vi "Prompt for Step--Update State Data.vi"(8 "error in (no error)":errorcluster, 9 "Data":variant, 10 "Argument":string, 11 "Keyboard Action in":refnum<class "Keyboard Action.lvclass">) -> (0 "error out":errorcluster, 3 "Keyboard Action out":refnum<class "Keyboard Action.lvclass">)   [LabVIEW 2020, in "MacroAssert.lvlib" / "Keyboard Action.lvclass"]
uses:
  Keyboard Action.lvclass
  Keyboard Action.lvclass/Keyboard Action.ctl
  Keyboard Action Type.ctl
  Action Step/Action Step.lvclass
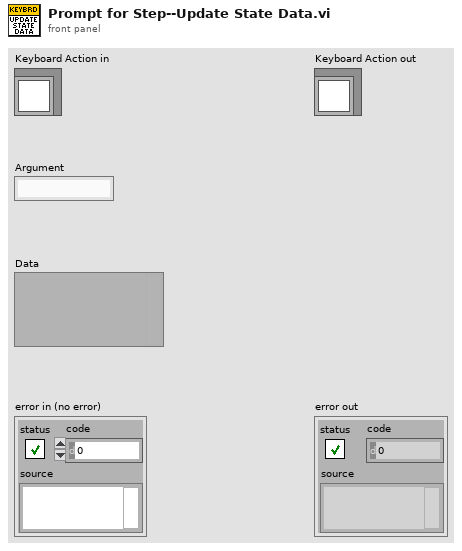
[diagram p1: front panel]
types:
  T1 = typedef "MacroAssert.lvlib/Keyboard Action.lvclass/Keyboard Action Type.ctl" = enum16{"Key Press", "Key Down", "Key Up"}
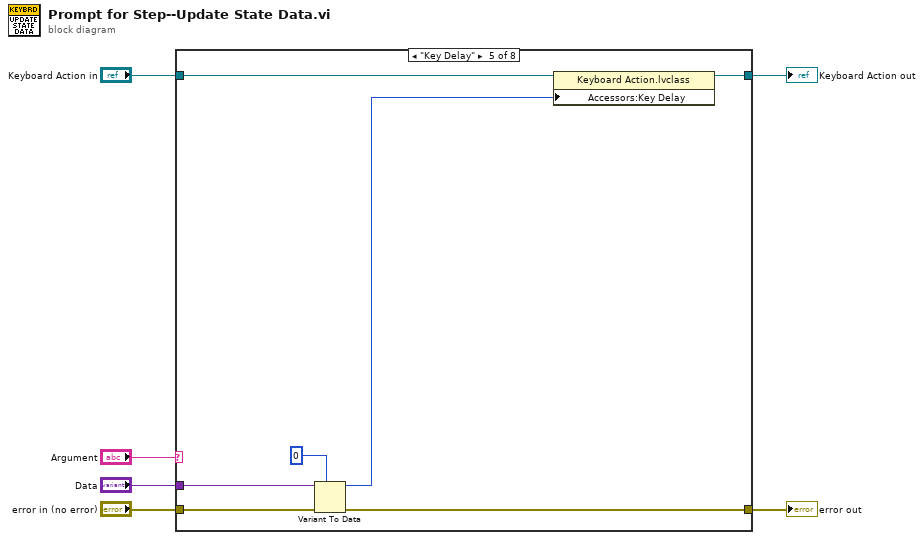
[diagram p0: block diagram]
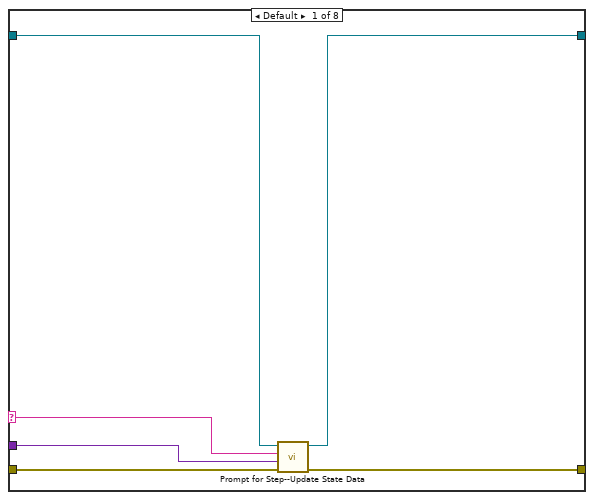
[diagram p2: hidden frame]
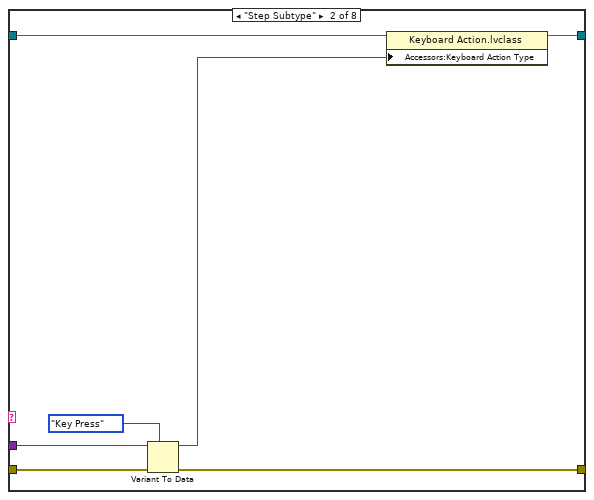
[diagram p3: hidden frame]
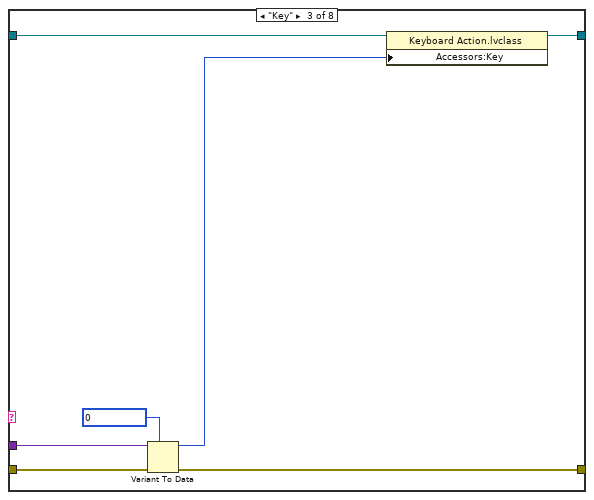
[diagram p4: hidden frame]
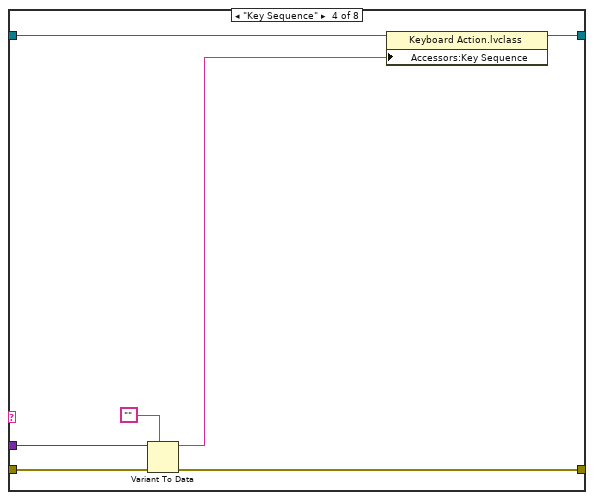
[diagram p5: hidden frame]
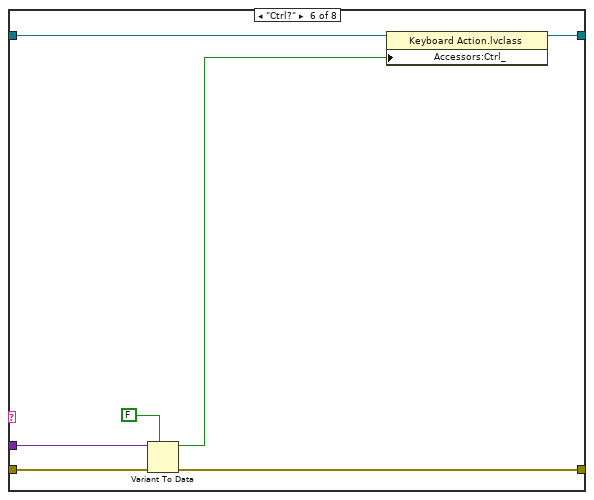
[diagram p6: hidden frame]
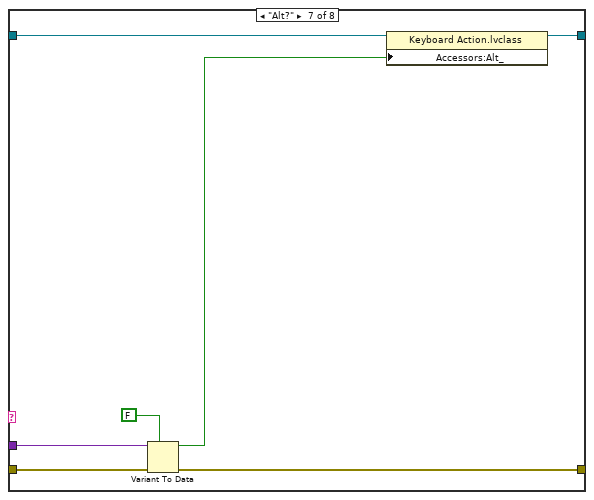
[diagram p7: hidden frame]
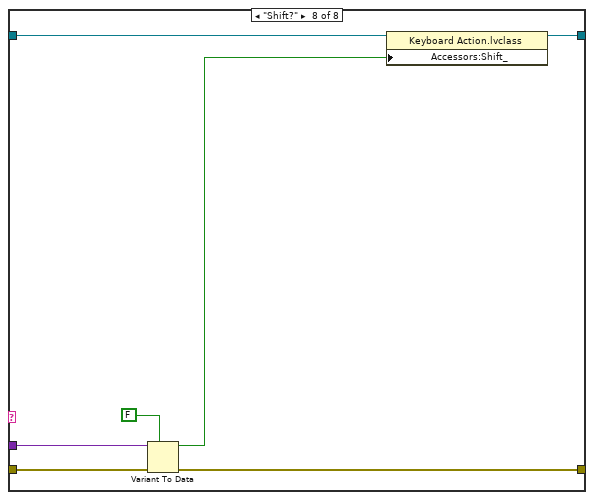
[diagram p8: hidden frame]
diagram:
  n1 = case shown="\"Key Delay\"" "Argument" {
    selector: "Argument" -> [w9 _ _ _ _ _ _ _]
    tunnel: "Keyboard Action in" -> [w8 w19 w26 w33 w40 w47 w54 w61]
    tunnel: "error in (no error)" -> [w12 w17 w24 w31 w38 w45 w52 w59]
    tunnel: [w7 w18 w25 w32 w39 w46 w53 w60] -> w3
    tunnel: [w11 w16 w23 w30 w37 w44 w51 w58] -> w5
    tunnel: "Data" -> [w10 w14 w22 w29 w36 w43 w50 w57]
    frame Default {
      n2 = call-parent "Prompt for Step--Update State Data.vi"("error in (no error)"=w12, "Data"=w10, "Argument"=w9, "Step in"=w8) -> ("error out"=w11:errorcluster, "Step out"=w7:refnum<class "Keyboard Action.lvclass">)  [unwired: 6 in]
    }
    frame "Step Subtype" {
      n3 = Variant To Data(error in=w17, type=Keyboard_Action_Type."Key Press" ("Keyboard Action Type"), Variant=w14) -> (data=w13:T1, error out=w16:errorcluster)
      n4 = property class="Keyboard Action.lvclass"(reference=w19, "Accessors:Keyboard Action Type"=w13) -> (reference out=w18:refnum<class "Keyboard Action.lvclass">)  [unwired: 1 in, 1 out]
    }
    frame "Key" {
      n5 = Variant To Data(error in=w24, type=u8 0 ("Key"), Variant=w22) -> (data=w20:u8, error out=w23:errorcluster)
      n6 = property class="Keyboard Action.lvclass"(reference=w26, "Accessors:Key"=w20) -> (reference out=w25:refnum<class "Keyboard Action.lvclass">)  [unwired: 1 in, 1 out]
    }
    frame "Key Sequence" {
      n7 = Variant To Data(error in=w31, type="", Variant=w29) -> (data=w28:string, error out=w30:errorcluster)
      n8 = property class="Keyboard Action.lvclass"(reference=w33, "Accessors:Key Sequence"=w28) -> (reference out=w32:refnum<class "Keyboard Action.lvclass">)  [unwired: 1 in, 1 out]
    }
    frame "Key Delay" {
      n9 = Variant To Data(error in=w38, type=0, Variant=w36) -> (data=w35:i32, error out=w37:errorcluster)
      n10 = property class="Keyboard Action.lvclass"(reference=w40, "Accessors:Key Delay"=w35) -> (reference out=w39:refnum<class "Keyboard Action.lvclass">)  [unwired: 1 in, 1 out]
    }
    frame "Ctrl?" {
      n11 = Variant To Data(error in=w45, type=FALSE, Variant=w43) -> (data=w42:bool, error out=w44:errorcluster)
      n12 = property class="Keyboard Action.lvclass"(reference=w47, "Accessors:Ctrl_"=w42) -> (reference out=w46:refnum<class "Keyboard Action.lvclass">)  [unwired: 1 in, 1 out]
    }
    frame "Alt?" {
      n13 = Variant To Data(error in=w52, type=FALSE, Variant=w50) -> (data=w49:bool, error out=w51:errorcluster)
      n14 = property class="Keyboard Action.lvclass"(reference=w54, "Accessors:Alt_"=w49) -> (reference out=w53:refnum<class "Keyboard Action.lvclass">)  [unwired: 1 in, 1 out]
    }
    frame "Shift?" {
      n15 = Variant To Data(error in=w59, type=FALSE, Variant=w57) -> (data=w56:bool, error out=w58:errorcluster)
      n16 = property class="Keyboard Action.lvclass"(reference=w61, "Accessors:Shift_"=w56) -> (reference out=w60:refnum<class "Keyboard Action.lvclass">)  [unwired: 1 in, 1 out]
    }
  }
  "error out" <- w5
  "Keyboard Action out" <- w3
